vi "通讯测试.vi"(3 "error in":errorcluster caption="错误输入") -> (5 "CMC":cluster{"表格控件":string[][], "啊打发":bool}, 6 "HVIL":T2 {"软件版本指示" items=["for 广汽新能源"=24004, "for 中航锂电"=25006, ""=0]}, 8 "error out":errorcluster caption="错误输出")   [LabVIEW 2020]
panel:
  # "F020  通讯测试"
  # "HVIL测试"
  # "Hz"
  # "判定：10±1Hz"
  # "判定：50±5%"
  # "%"
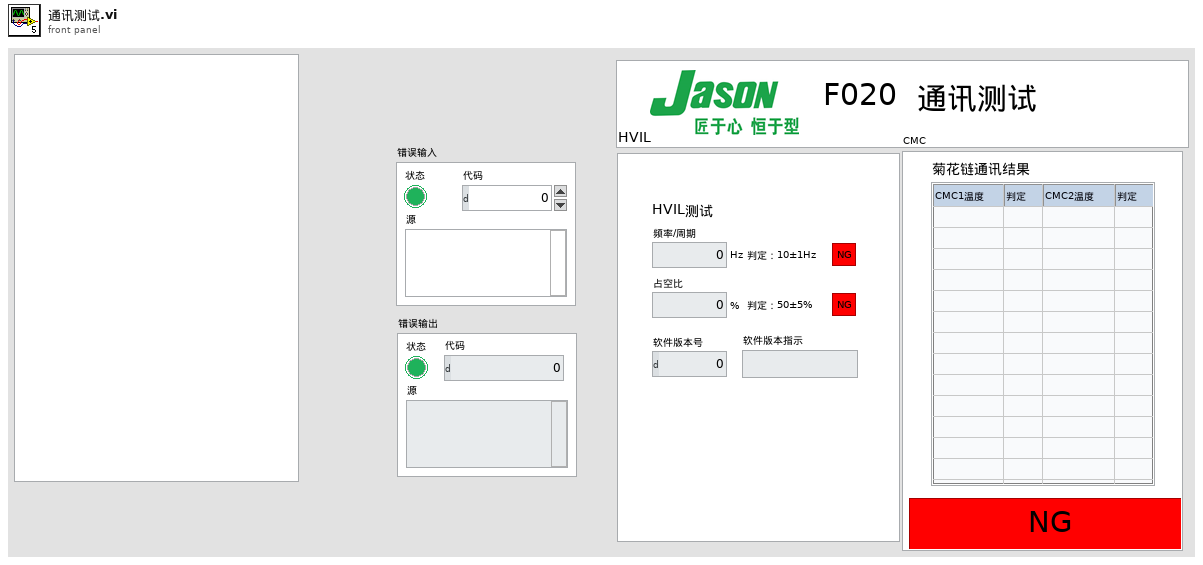
[diagram p1: front panel]
types:
  T1 = typedef "软件版本指示.ctl" = u32
  T2 = cluster{"占空比":u32, "频率/周期":u32, "软件版本号":u32, "频率判定":bool, "占空比判定":bool, "软件版本指示":T1}
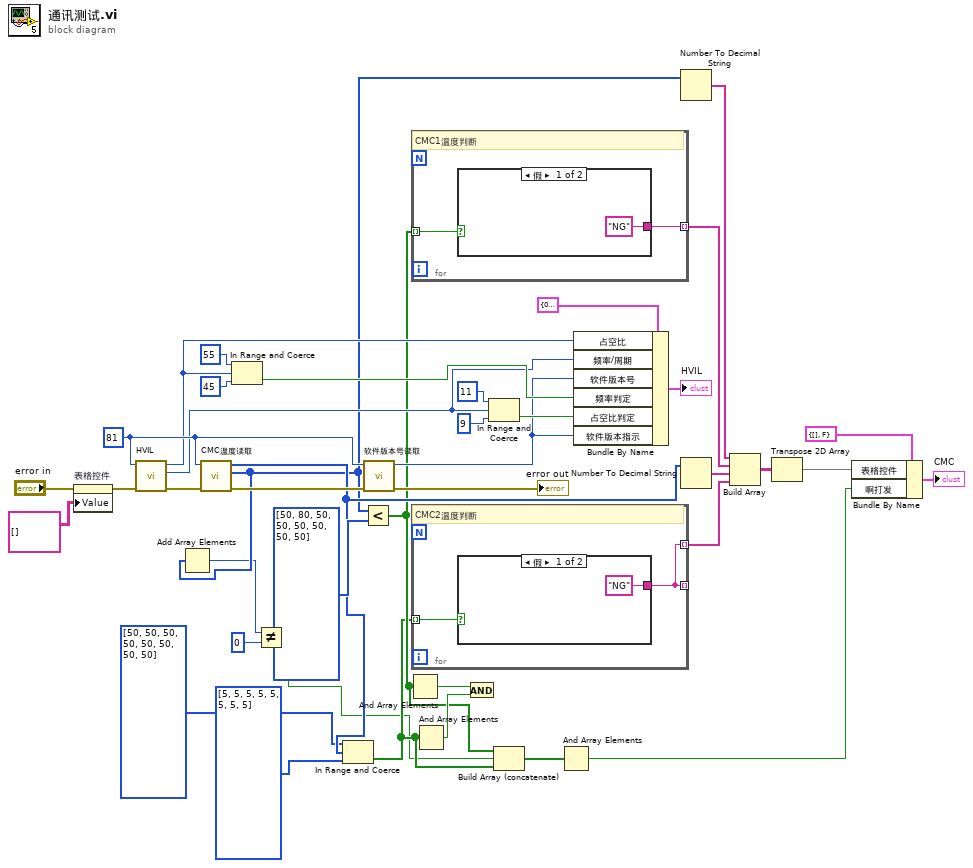
[diagram p0: block diagram]
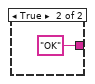
[diagram p2: hidden frame]
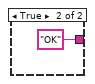
[diagram p3: hidden frame]
diagram:
  w38 = u16 81 ("Channel")
  n1 = property on="表格控件" class="Tbl (严格)"(error in="error in", "Value"=string[][] [] ("表格控件")) -> (error out=w23:errorcluster)  [unwired: 1 in, 1 out]
  n2 = call "HVIL.vi"("error in"=w23, "Channel"=w38) -> ("error out"=w29:errorcluster, "频率/周期"=w12:u32, "占空比"=w20:u32)  [unwired: 7 in]
  n3 = call "CMC温度读取.vi"("error in"=w29, "Channel"=w38) -> ("error out"=w40:errorcluster, "CMC1温度"=w3:i32[], "CMC2温度"=w11:i32[])  [unwired: 7 in]
  n4 = Add Array Elements(numeric array=w3) -> (sum=w2:i32)
  n5 = In Range and Coerce(upper limit=u32 55 ("上限"), x=w20, lower limit=u32 45 ("下限")) -> (In Range?=w19:bool)  [unwired: 1 out]
  n6 = Not Equal?(x=w2, y=0) -> (x != y?=w6:bool)
  n7 = In Range and Coerce(upper limit=i32[] [50, 50, 50, 50, 50, 50, 50, 50], x=w11, lower limit=i32[] [5, 5, 5, 5, 5, 5, 5, 5]) -> (In Range?=w7:bool[])  [unwired: 1 out]
  n8 = Less?(x=w3, y=i32[] [50, 80, 50, 50, 50, 50, 50, 50]) -> (x < y?=w8:bool[])
  n9 = call "软件版本号读取.vi"("error in"=w40, "Channel"=w38) -> ("error out"=→"error out":errorcluster, "软件版本号"=w13:u32)  [unwired: 8 in]
  n10 = And Array Elements(Boolean array=w8) -> (logical AND=w31:bool)
  n11 = for {
    tunnel: w8 -> [w42] mode=indexing
    tunnel: [w41] -> w35 mode=indexing
    # "CMC1温度判断"
    n12 = case shown="假" w42 {
      tunnel: ["NG" "OK"] -> w41
      frame False {
      }
      frame True {
      }
    }
  }
  n13 = for {
    tunnel: w7 -> [w46] mode=indexing
    tunnel: [w45] -> _ mode=indexing
    tunnel: [w45] -> w33 mode=indexing
    # "CMC2温度判断"
    n14 = case shown="假" w46 {
      tunnel: ["NG" "OK"] -> w45
      frame False {
      }
      frame True {
      }
    }
  }
  n15 = And Array Elements(Boolean array=w7) -> (logical AND=w30:bool)
  n16 = And(x=w31, y=w30) -> ()  [unwired: 1 out]
  n17 = In Range and Coerce(upper limit=u32 11 ("上限"), x=w12, lower limit=u32 9 ("下限")) -> (In Range?=w18:bool)  [unwired: 1 out]
  n18 = Build Array (concatenate)(w8, w6, w7) -> (w5:bool[])
  n19 = And Array Elements(Boolean array=w5) -> (logical AND=w4:bool)
  n20 = Bundle By Name(cluster=T2 {"占空比"=0, "频率/周期"=0, "软件版本号"=0, "频率判定"=FALSE, "占空比判定"=FALSE, "软件版本指示"=0}, "占空比"=w20, "频率/周期"=w12, "软件版本号"=w13, "频率判定"=w19, "占空比判定"=w18, "软件版本指示"=w13) -> (→"HVIL":T2)
  n21 = Number To Decimal String(number=w3) -> (decimal integer string=w36:string[])  [unwired: 1 in]
  n22 = Number To Decimal String(number=w11) -> (decimal integer string=w34:string[])  [unwired: 1 in]
  n23 = Build Array(w36, w35, w34, w33) -> (w32:string[][])
  n24 = Transpose 2D Array(2D array=w32) -> (transposed array=w14:string[][])
  n25 = Bundle By Name(cluster=cluster{"表格控件":string[][], "啊打发":bool} {"表格控件"=[], "啊打发"=FALSE} ("CMC"), "表格控件"=w14, "啊打发"=w4) -> (→"CMC":cluster{"表格控件":string[][], "啊打发":bool})
